vi "client.vi"() -> ()   [LabVIEW 2019]
uses:
  Generated_client/RPC Messages/Greeter_req.ctl
  Generated_client/RPC Messages/Greeter_MessageA.ctl
  Generated_client/RPC Messages/Greeter_req_req_oneof/Greeter_req_req_oneof.lvclass
  Generated_client/RPC Messages/Greeter_req_req_oneof/Greeter_req_req_oneof.lvclass/Greeter_req_req_oneof.ctl
  Generated_client/RPC Messages/Greeter_res_res_oneof/Greeter_res_res_oneof.lvclass/Greeter_res_res_oneof.ctl
  Generated_client/Generated_client.lvlib
  Generated_client/RPC Messages/Greeter_res_res_oneof/Greeter_res_res_oneof.lvclass
panel:
  out "res_name":string
  out "res_id":i32
  out "res_data_a1":string
  out "res_latitude":i32
  in  "req_latitude":i32=101
  in  "data_a1":string="da"
  in  "req_id":i32=111
  in  "req_name":string="daa"
  in  "req_oneof":enum16{"req_id", "req_name", ""}(ring)
  out "error out":errorcluster
  in  "error in":errorcluster
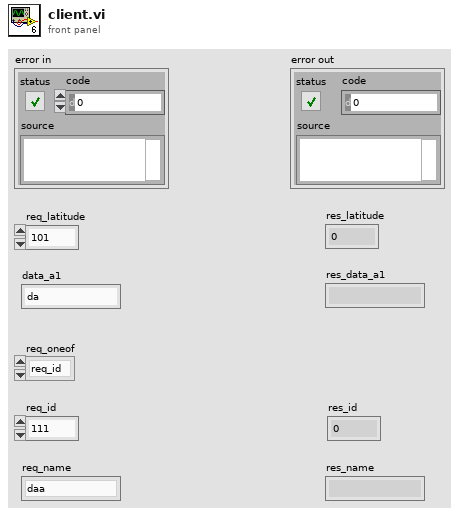
[diagram p1: front panel]
types:
  T1 = typedef "Generated_client.lvlib/Greeter_MessageA.ctl" = cluster{"data_a1":string}
  T2 = typedef "Generated_client.lvlib/Greeter_req.ctl" = cluster{"req_latitude":i32, "message_a":T1, "Greeter_req_req_oneof":refnum<class "Greeter_req_req_oneof.lvclass">}
  T3 = typedef "grpc-lvsupport-release.lvlib/grpcId.ctl" = u64
  T4 = typedef "Generated_client.lvlib/Greeter_res.ctl" = cluster{"res_latitude":i32, "Greeter_res_res_oneof":refnum<class "Greeter_res_res_oneof.lvclass">, "message_a":T1}
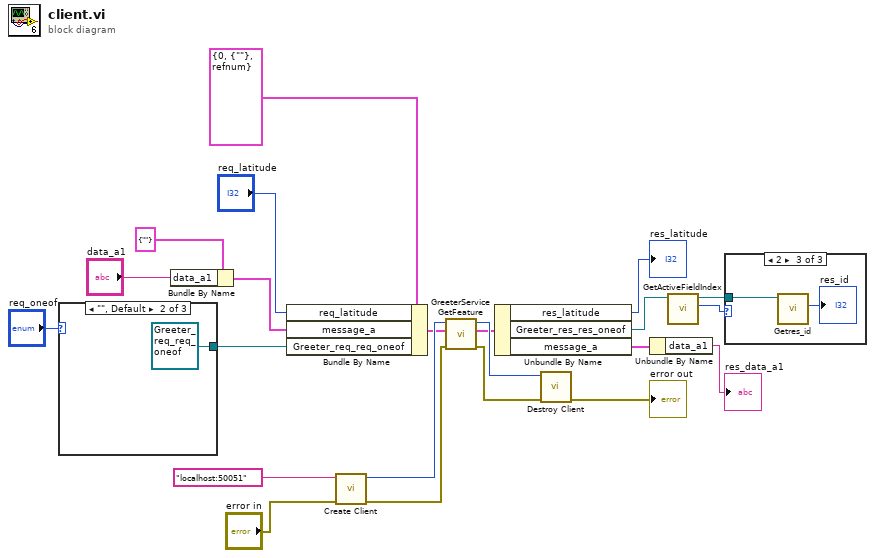
[diagram p0: block diagram]
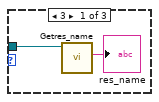
[diagram p2: hidden frame]
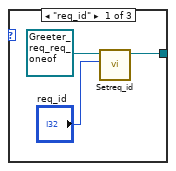
[diagram p4: hidden frame]
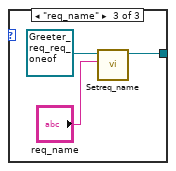
[diagram p5: hidden frame]
diagram:
  n1 = case shown="\"\", Default" "req_oneof" {
    tunnel: [w23 refnum<class "Greeter_req_req_oneof.lvclass"> refnum ("OneOfTemplate out") w27] -> w14
    frame "req_id" {
      n2 = call "Setreq_id.vi"("Set_Val"="req_id", "OneOfTemplate in"=refnum<class "Greeter_req_req_oneof.lvclass"> refnum) -> ("OneOfTemplate out"=w23:refnum<class "Greeter_req_req_oneof.lvclass">)  [unwired: 8 in, 1 out]
    }
    frame "", Default {
    }
    frame "req_name" {
      n3 = call "Setreq_name.vi"("Set_Val"="req_name", "OneOfTemplate in"=refnum<class "Greeter_req_req_oneof.lvclass"> refnum) -> ("OneOfTemplate out"=w27:refnum<class "Greeter_req_req_oneof.lvclass">)  [unwired: 8 in, 1 out]
    }
  }
  n4 = Bundle By Name(cluster=T1 {"data_a1"=""} ("Greeter_MessageA"), "data_a1"="data_a1") -> (w10:T1)
  n5 = Bundle By Name(cluster=T2 {"req_latitude"=0, "message_a"={"data_a1"=""}, "Greeter_req_req_oneof"=refnum} ("Greeter_req"), "req_latitude"="req_latitude", "message_a"=w10, "Greeter_req_req_oneof"=w14) -> (w8:T2)
  n6 = call "Create Client.vi"("error in"="error in", "address"="localhost:50051") -> ("error out"=w20:errorcluster, "gRPC ID Out"=w22:T3)  [unwired: 8 in]
  n7 = call "GreeterService GetFeature.vi"("error in"=w20, "Request Data"=w8, "gRPC ID"=w22) -> ("error out"=w19:errorcluster, "Response Data"=w7:T4, "gRPC ID out"=w21:T3)  [unwired: 6 in]
  n8 = Unbundle By Name(w7) -> ("res_latitude"=→"res_latitude":i32, "Greeter_res_res_oneof"=w3:refnum<class "Greeter_res_res_oneof.lvclass">, "message_a"=w5:T1)
  n9 = call "Destroy Client.vi"("error in"=w19, "gRPC ID"=w21) -> ("error out"=→"error out":errorcluster)  [unwired: 9 in]
  n10 = Unbundle By Name(w5) -> ("data_a1"=→"res_data_a1":string)
  n11 = call "GetActiveFieldIndex.vi"("OneOfTemplate in"=w3) -> ("Active Field Index"=w1:i32, "OneOfTemplate out"=w2:refnum<class "Greeter_res_res_oneof.lvclass">)  [unwired: 8 in, 1 out]
  n12 = case shown="2" w1 {
    tunnel: w2 -> [w31 _ w33]
    frame 3 {
      n13 = call "Getres_name.vi"("OneOfTemplate in"=w31) -> ("Get_Val"=→"res_name":string)  [unwired: 8 in, 2 out]
    }
    frame 0, Default {
    }
    frame 2 {
      n14 = call "Getres_id.vi"("OneOfTemplate in"=w33) -> ("Get_Val"=→"res_id":i32)  [unwired: 8 in, 2 out]
    }
  }
